vi "Get Scope Time Array from Waveform.vi"(8 "error in (no error)":errorcluster, 9 "Average Number of Points":dbl format="%#_13g", 10 "Record Length (points)":i32, 11 "Waveform Data":waveform(dbl)) -> (0 "error out":errorcluster, 3 "Time Axis":dbl[](array[numeric]))   [LabVIEW 2017, in "File IO.lvlib"]
uses:
  File IO.lvlib
  <vilib>/Analysis/2dsp.llb/Decimate (single shot, DBL).vi
  <vilib>/Analysis/NI_AALPro.lvlib
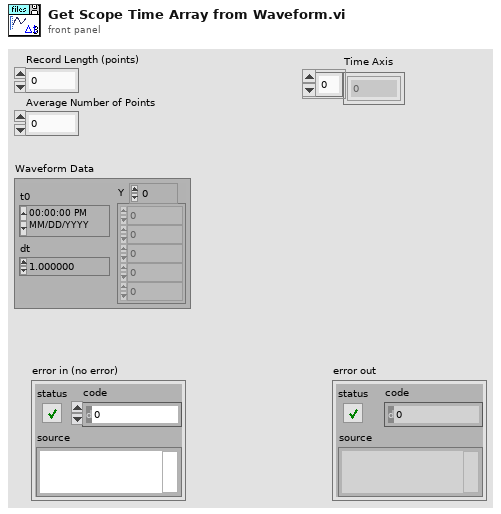
[diagram p1: front panel]
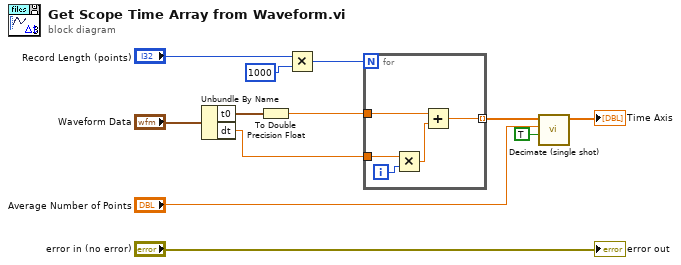
[diagram p0: block diagram]
diagram:
  n1 = Unbundle By Name("Waveform Data") -> ("t0"=w9:timestamp, "dt"=w8:dbl)
  n2 = To Double Precision Float(number=w9) -> (double precision float=w12:dbl)
  n3 = Multiply(x="Record Length (points)", y=1000) -> (x*y=w2:i32)
  n4 = for {
    N: w2 -> [_]
    tunnel: w12 -> [w17]
    tunnel: w8 -> [w15]
    tunnel: [w13] -> w11 mode=indexing
    i -> [w16]
    n5 = Multiply(x=w15, y=w16) -> (x*y=w14:dbl)
    n6 = Add(x=w17, y=w14) -> (x+y=w13:dbl)
  }
  n7 = call-poly <vilib>:"Decimate (single shot).vi"("averaging"=TRUE, "decimating factor"="Average Number of Points", "X"=w11) -> ("Decimated Array"=→"Time Axis":dbl[])  [unwired: 7 in, 1 out]
  "error out" <- "error in (no error)"
